vi "Build Cycle Instructions.vi"(4 "FPGA":T6, 5 "DUT Mode":enum32{"All", "Single"}(radio), 6 "Select Cycle Pattern":enum16{"Pattern 1", "Pattern 2"}(ring), 8 "error in":errorcluster, 9 "Cycle Pairs":T5[](array[typedef])=[{"G1 Ch (0-5)"=1, "G2 Ch (0-5)"=0, "En"=TRUE}, {"G1 Ch (0-5)"=3, "G2 Ch (0-5)"=2, "En"=TRUE}, {"G1 Ch (0-5)"=4, "G2 Ch (0-5)"=5, "En"=TRUE}] {"G2 Ch (0-5)" max=5 step=1 format="Ch %.0f"; "G1 Ch (0-5)" max=5 step=1 format="Ch %.0f"}, 11 "System In":T1={"I2C Monitor"=TRUE, "SRL Cyle"=TRUE, "DAC Vout (V)"=0.0, "DUT Ch Idx (0-5)"=0, "Cycle Instructions"=[], "Vout 1 (V)"=0.0, "Delay 1 (s)"=0.0, "Number of pairs"=2, "Delay 2 (s)"=0.0, "Data Out (14-bit)"=0, "DUT"=enum."DUT 01", "Vout 2 (V)"=0.0, "Cycle Scheme"=enum."All Channels"} {"Vout 2 (V)" format="%.3f V"; "Data Out (14-bit)" max=5 step=1 format="0x%04x"; "Delay 2 (s)" format="%#_4ps"; "Number of pairs" min=1 max=4 step=1; "Delay 1 (s)" format="%#_4ps"; "Vout 1 (V)" format="%.3f V"; "Cycle Instructions"."Post CMD Delay (s)" format="%#_4ps"; "Cycle Instructions"."DAC Vout (V)" format="%.3f V"; "Cycle Instructions"."Dev Ch Idx (0-5)" max=5 step=1 format="Ch %d"; "DUT Ch Idx (0-5)" max=5 step=1; "DAC Vout (V)" format="%.3f V"}) -> (0 "error out":errorcluster, 2 "Dev Idx (0-5)":u32, 3 "System Out":T1={"I2C Monitor"=TRUE, "SRL Cyle"=TRUE, "DAC Vout (V)"=0.0, "DUT Ch Idx (0-5)"=0, "Cycle Instructions"=[], "Vout 1 (V)"=0.0, "Delay 1 (s)"=0.0, "Number of pairs"=2, "Delay 2 (s)"=0.0, "Data Out (14-bit)"=0, "DUT"=enum."DUT 01", "Vout 2 (V)"=0.0, "Cycle Scheme"=enum."All Channels"} {"Vout 2 (V)" format="%.3f V"; "Data Out (14-bit)" max=5 step=1 format="0x%04x"; "Delay 2 (s)" format="%#_4ps"; "Number of pairs" min=1 max=4 step=1; "Delay 1 (s)" format="%#_4ps"; "Vout 1 (V)" format="%.3f V"; "Cycle Instructions"."Post CMD Delay (s)" format="%#_4ps"; "Cycle Instructions"."DAC Vout (V)" format="%.3f V"; "Cycle Instructions"."Dev Ch Idx (0-5)" max=5 step=1 format="Ch %d"; "DUT Ch Idx (0-5)" max=5 step=1; "DAC Vout (V)" format="%.3f V"})   [LabVIEW 2017, in "Host SRL.lvlib"]
uses:
  Host SRL.lvlib
  Type Defs/Cycle Instruction Cluster.ctl
  Type Defs/WSVCAP SHL FPGA Enum.ctl
  Type Defs/Cycle Pair Cluster.ctl
  Type Defs/WSVCAP SHL Tester System Cluster.ctl
  Type Defs/WSVCAP SHL DUT Number Enum.ctl
  Type Defs/Cycle Scheme Enum.ctl
panel:
  out "Cycle Instructions":T2[](array[typedef]) {"Post CMD Delay (s)" format="%#_4ps"; "DAC Vout (V)" format="%.3f V"; "Dev Ch Idx (0-5)" max=5 step=1 format="Ch %d"}
  # "Group 1"
  # "Group 2"
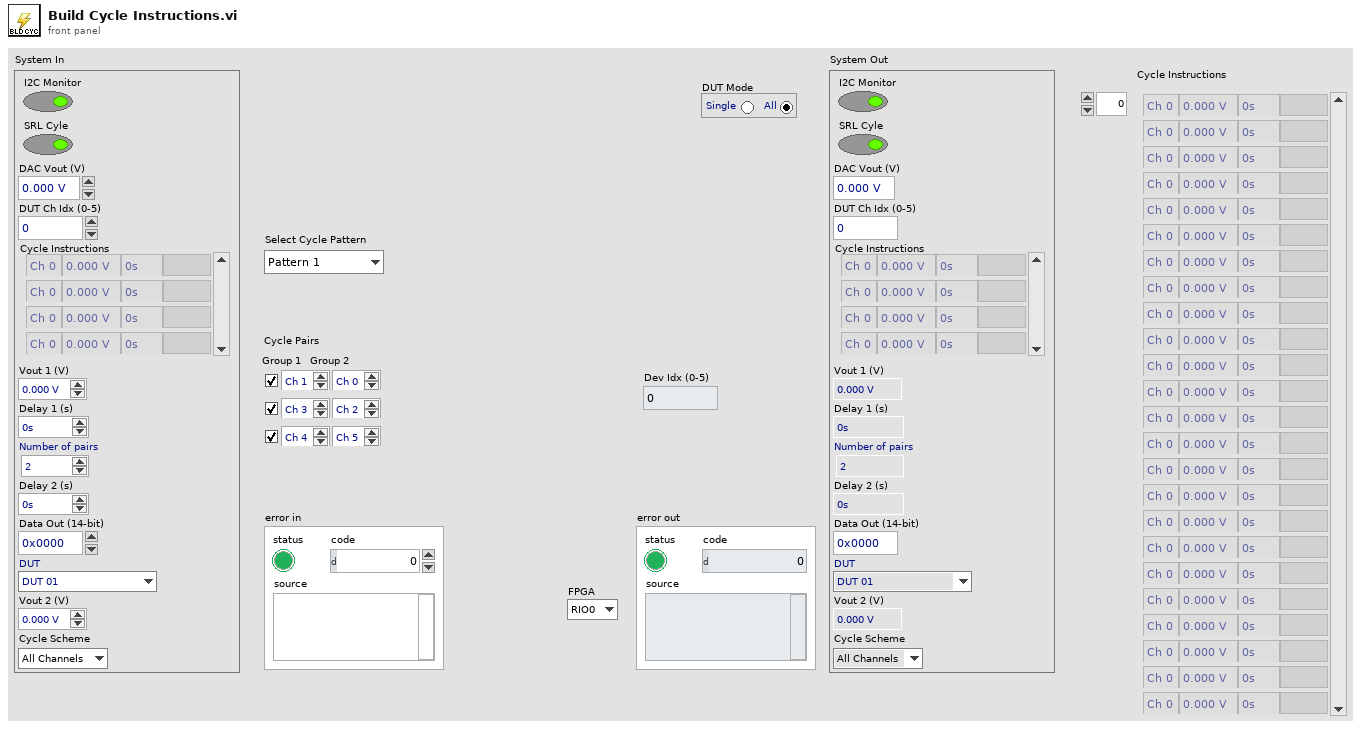
[diagram p1: front panel]
types:
  T1 = typedef "WSVCAP SHL Tester System Cluster.ctl" = cluster{"I2C Monitor":bool, "SRL Cyle":bool, "DAC Vout (V)":dbl, "DUT Ch Idx (0-5)":u32, "Cycle Instructions":T2[], "Vout 1 (V)":dbl, "Delay 1 (s)":dbl, "Number of pairs":i32, "Delay 2 (s)":dbl, "Data Out (14-bit)":u16, "DUT":T3, "Vout 2 (V)":dbl, "Cycle Scheme":T4}
  T2 = typedef "Host SRL.lvlib/Cycle Instruction Cluster.ctl" = cluster{"Dev Ch Idx (0-5)":u32, "DAC Vout (V)":dbl, "Post CMD Delay (s)":dbl, "Raw CMD":string}
  T3 = typedef "WSVCAP SHL DUT Number Enum.ctl" = enum16{"DUT 01", "DUT 02", "DUT 03", "DUT 04", "DUT 05", "DUT 06", "DUT 07", "DUT 08", "DUT 09", "DUT 10", "DUT 11", "DUT 12", "DUT 13", "DUT 14", "DUT 15", "DUT 16", "DUT 17", "DUT 18", "DUT 19", "DUT 20", "DUT 21", "DUT 22", "DUT 23", "DUT 24"}
  T4 = typedef "Cycle Scheme Enum.ctl" = enum16{"All Channels", "By Group"}
  T5 = typedef "Host SRL.lvlib/Cycle Pair Cluster.ctl" = cluster{"G1 Ch (0-5)":u32, "G2 Ch (0-5)":u32, "En":bool}
  T6 = typedef "WSVCAP SHL FPGA Enum.ctl" = enum16{"RIO0", "RIO1"}
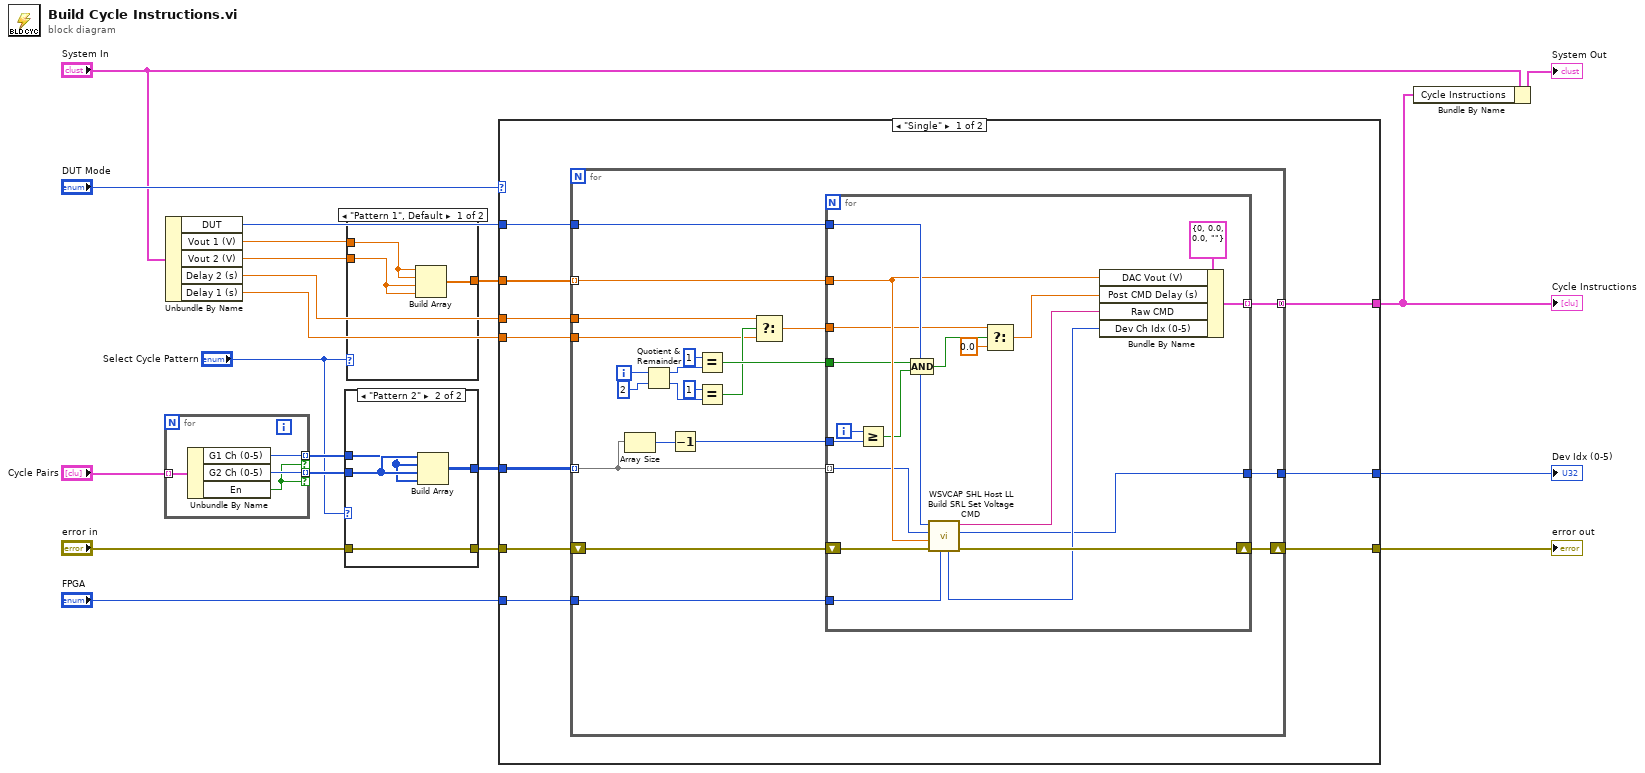
[diagram p0: block diagram]
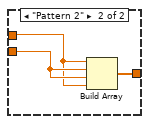
[diagram p2: hidden frame]
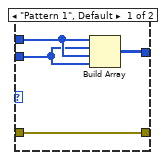
[diagram p3: hidden frame]
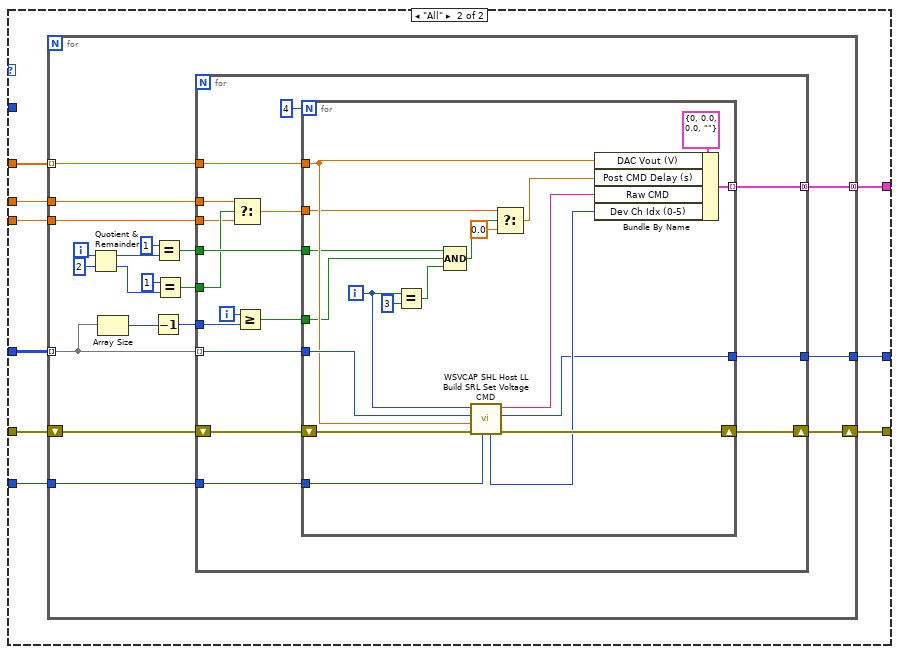
[diagram p4: hidden frame]
diagram:
  n1 = for {
    tunnel: "Cycle Pairs" -> [w24] mode=indexing
    tunnel: [w23] -> w4 mode=indexing if=w21
    tunnel: [w22] -> w5 mode=indexing if=w21
    n2 = Unbundle By Name(w24) -> ("G1 Ch (0-5)"=w23:u32, "G2 Ch (0-5)"=w22:u32, "En"=w21:bool)
  }
  n3 = Unbundle By Name("System In") -> ("DUT"=w10:T3, "Vout 1 (V)"=w6:dbl, "Vout 2 (V)"=w7:dbl, "Delay 2 (s)"=w9:dbl, "Delay 1 (s)"=w8:dbl)
  n4 = case shown="\"Pattern 2\"" "Select Cycle Pattern" {
    tunnel: [w25 w32] -> w16
    tunnel: w5 -> [w26 w31]
    tunnel: w4 -> [w27 w30]
    tunnel: [w28 w29] -> w2
    tunnel: "error in" -> [w28 w29]
    frame "Pattern 1", Default {
      n5 = Build Array(w27, w26, w27, w26) -> (w25:u32[][])
    }
    frame "Pattern 2" {
      n6 = Build Array(w31, w30, w31, w30) -> (w32:u32[][])
    }
  }
  n7 = case shown="\"Pattern 1\", Default" "Select Cycle Pattern" {
    tunnel: [w35 w38] -> w15
    tunnel: w7 -> [w33 w37]
    tunnel: w6 -> [w34 w36]
    frame "Pattern 1", Default {
      n8 = Build Array(w34, w34, w33, w33) -> (w35:dbl[])
    }
    frame "Pattern 2" {
      n9 = Build Array(w36, w37, w37, w36) -> (w38:dbl[])
    }
  }
  n10 = case shown="\"Single\"" "DUT Mode" {
    tunnel: [w48 w97] -> w11
    tunnel: w10 -> [w47 _]
    tunnel: "FPGA" -> [w46 w96]
    tunnel: w2 -> [w45 w95]
    tunnel: [w44 w94] -> w18
    tunnel: [w43 w89] -> w17
    tunnel: w16 -> [w42 w92]
    tunnel: w15 -> [w41 w93]
    tunnel: w8 -> [w40 w91]
    tunnel: w9 -> [w39 w90]
    frame "Single" {
      n11 = for {
        tunnel: [w69] -> w48 mode=concatenating
        tunnel: w47 -> [w68]
        tunnel: w46 -> [w67]
        shift-right: [w65] -> w44
        shift-left: w45 -> [w66]
        tunnel: [w64] -> w43
        tunnel: w42 -> [w62] mode=indexing
        tunnel: w41 -> [w63] mode=indexing
        tunnel: w40 -> [w50]
        tunnel: w39 -> [w51]
        i -> [w59]
        n12 = Array Size(array=w62) -> (size(s)=w61:i32)
        n13 = Quotient & Remainder(x=w59, y=2) -> (x-y*floor(x/y)=w57:i32, floor(x/y)=w53:i32)
        n14 = Decrement(x=w61) -> (x-1=w60:i32)
        n15 = Equal?(x=1, y=w57) -> (x = y?=w55:bool)
        n16 = Equal?(x=1, y=w53) -> (x = y?=w52:bool)
        n17 = Select(t=w51, s=w52, f=w50) -> (s? t:f=w49:dbl)
        n18 = for {
          tunnel: [w87] -> w69 mode=indexing
          tunnel: w68 -> [w86]
          tunnel: w67 -> [w85]
          tunnel: [w81] -> w64
          shift-right: [w83] -> w65
          shift-left: w66 -> [w84]
          tunnel: w62 -> [w78] mode=indexing
          tunnel: w63 -> [w79]
          tunnel: w60 -> [w76]
          tunnel: w49 -> [w73]
          tunnel: w55 -> [w72]
          i -> [w77]
          n19 = Greater Or Equal?(x=w77, y=w76) -> (x >= y?=w71:bool)
          n20 = Compound Arithmetic op=AND(w72, w71) -> (w70:bool)
          n21 = call "WSVCAP SHL Host LL Build SRL Set Voltage CMD.vi"("FPGA (Required for Vref = -1)"=w85, "error in (no error)"=w84, "Voltage (-1: Use Data Out)"=w79, "Channel (0-5)"=w78, "DUT"=w86) -> ("error out"=w83:errorcluster, "Dev Idx (0-5)"=w81:u32, "Raw CMD [Str]"=w80:string, "Device Ch Idx (0-31)"=w82:u32)  [unwired: 2 in, 1 out]
          n22 = Select(t=w73, s=w70, f=0.0) -> (s? t:f=w75:dbl)
          n23 = Bundle By Name(cluster=T2 {"Dev Ch Idx (0-5)"=0, "DAC Vout (V)"=0.0, "Post CMD Delay (s)"=0.0, "Raw CMD"=""} ("Cycle Instruction Cluster"), "DAC Vout (V)"=w79, "Post CMD Delay (s)"=w75, "Raw CMD"=w80, "Dev Ch Idx (0-5)"=w82) -> (w87:T2)
        }
      }
    }
    frame "All" {
      n24 = for {
        tunnel: [w116] -> w97 mode=concatenating
        tunnel: w96 -> [w115]
        shift-right: [w113] -> w94
        shift-left: w95 -> [w114]
        tunnel: w93 -> [w112] mode=indexing
        tunnel: w92 -> [w104] mode=indexing
        tunnel: w91 -> [w111]
        tunnel: w90 -> [w99]
        tunnel: [w98] -> w89
        i -> [w107]
        n25 = Quotient & Remainder(x=w107, y=2) -> (x-y*floor(x/y)=w108:i32, floor(x/y)=w101:i32)
        n26 = Array Size(array=w104) -> (size(s)=w105:i32)
        n27 = Decrement(x=w105) -> (x-1=w103:i32)
        n28 = Equal?(x=1, y=w108) -> (x = y?=w106:bool)
        n29 = Equal?(x=1, y=w101) -> (x = y?=w100:bool)
        n30 = for {
          tunnel: [w132] -> w116 mode=concatenating
          tunnel: w115 -> [w130]
          shift-right: [w128] -> w113
          shift-left: w114 -> [w129]
          tunnel: w112 -> [w127]
          tunnel: w104 -> [w126] mode=indexing
          tunnel: w111 -> [w119]
          tunnel: w106 -> [w125]
          tunnel: w103 -> [w123]
          tunnel: w100 -> [w121]
          tunnel: w99 -> [w120]
          tunnel: [w117] -> w98
          i -> [w124]
          n31 = Select(t=w120, s=w121, f=w119) -> (s? t:f=w118:dbl)
          n32 = Greater Or Equal?(x=w124, y=w123) -> (x >= y?=w122:bool)
          n33 = for {
            N: 4 -> [_]
            tunnel: [w150] -> w132 mode=indexing
            tunnel: w130 -> [w149]
            shift-right: [w147] -> w128
            shift-left: w129 -> [w148]
            tunnel: w127 -> [w143]
            tunnel: w126 -> [w144]
            tunnel: w118 -> [w136]
            tunnel: w125 -> [w135]
            tunnel: w122 -> [w134]
            tunnel: [w133] -> w117
            i -> [w137]
            n34 = Equal?(x=w137, y=3) -> (x = y?=w140:bool)
            n35 = Compound Arithmetic op=AND(w135, w134, w140) -> (w139:bool)
            n36 = call "WSVCAP SHL Host LL Build SRL Set Voltage CMD.vi"("FPGA (Required for Vref = -1)"=w149, "error in (no error)"=w148, "Voltage (-1: Use Data Out)"=w143, "Channel (0-5)"=w144, "DUT"=w137) -> ("error out"=w147:errorcluster, "Dev Idx (0-5)"=w133:u32, "Raw CMD [Str]"=w146:string, "Device Ch Idx (0-31)"=w145:u32)  [unwired: 2 in, 1 out]
            n37 = Select(t=w136, s=w139, f=0.0) -> (s? t:f=w138:dbl)
            n38 = Bundle By Name(cluster=T2 {"Dev Ch Idx (0-5)"=0, "DAC Vout (V)"=0.0, "Post CMD Delay (s)"=0.0, "Raw CMD"=""} ("Cycle Instruction Cluster"), "DAC Vout (V)"=w143, "Post CMD Delay (s)"=w138, "Raw CMD"=w146, "Dev Ch Idx (0-5)"=w145) -> (w150:T2)
          }
        }
      }
    }
  }
  "Cycle Instructions" <- w11
  "error out" <- w18
  "Dev Idx (0-5)" <- w17
  n39 = Bundle By Name(cluster="System In", "Cycle Instructions"=w11) -> (→"System Out":T1)
